vi "Place-cursor.vi"(0 "star X":i16, 1 "GuidePixScale":dbl=0.32, 2 "star Y":i16, 3 "Angle":dbl=0.707, 5 "GuideGraph":refnum<vi>) -> (6 "RA cursor":dbl, 10 "DEC cursor":dbl)   [LabVIEW 2011]
panel:
  in  "camYsize":dbl=480.0
  in  "camXsize":dbl=640.0
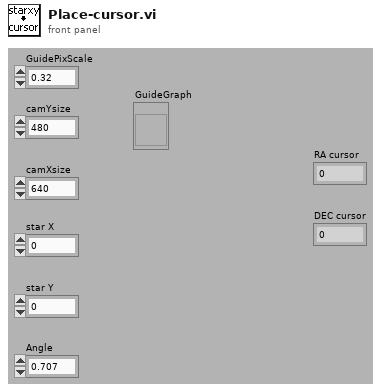
[diagram p1: front panel]
types:
  T1 = typedef "LVRangeTypeDef.ctl" = cluster{"Minimum":dbl, "Maximum":dbl, "Increment":dbl, "Minor Increment":dbl, "Start":dbl}
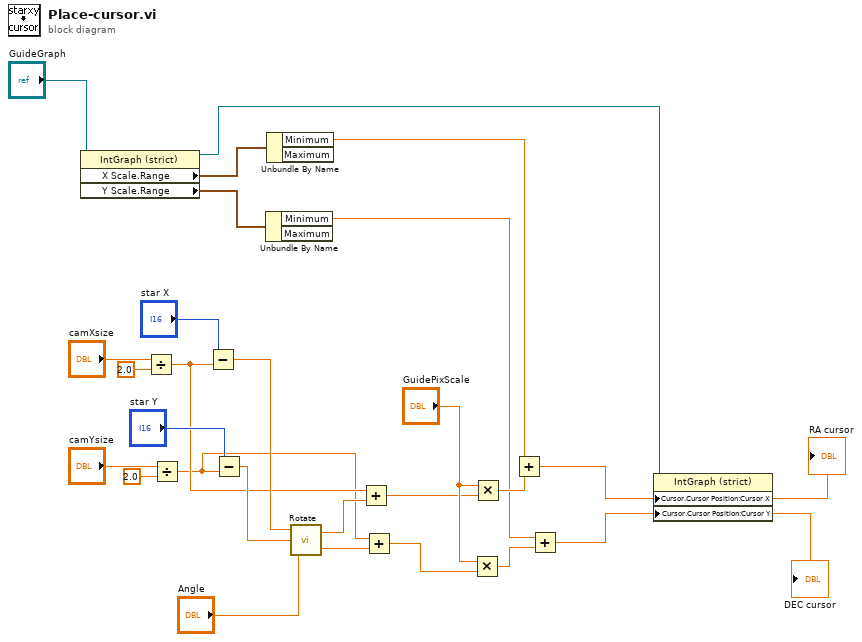
[diagram p0: block diagram]
diagram:
  n1 = property on="Property Node" class="IntGraph (strict)"(reference="GuideGraph") -> (reference out=w10:refnum<vi>, "X Scale.Range"=w18:T1, "Y Scale.Range"=w17:T1)  [unwired: 1 in, 1 out]
  n2 = Divide(x="camXsize", y=2.0) -> (x/y=w7:dbl)
  n3 = Divide(x="camYsize", y=2.0) -> (x/y=w5:dbl)
  n4 = Subtract(x="star X", y=w7) -> (x-y=w19:dbl)
  n5 = Subtract(x="star Y", y=w5) -> (x-y=w20:dbl)
  n6 = Unbundle By Name(w17) -> ("Minimum"=w12:dbl)  [unwired: 1 out]
  n7 = Unbundle By Name(w18) -> ("Minimum"=w13:dbl)  [unwired: 1 out]
  n8 = call "Rotate.vi"("Angle(rad)"="Angle", "Y"=w20, "X"=w19) -> ("rotY"=w4:dbl, "rotX"=w6:dbl)
  n9 = Add(x=w7, y=w6) -> (x+y=w3:dbl)
  n10 = Add(x=w5, y=w4) -> (x+y=w2:dbl)
  n11 = Multiply(x="GuidePixScale", y=w2) -> (x*y=w15:dbl)
  n12 = Multiply(x="GuidePixScale", y=w3) -> (x*y=w16:dbl)
  n13 = Add(x=w13, y=w16) -> (x+y=w9:dbl)
  "RA cursor" <- w9
  n14 = Add(x=w12, y=w15) -> (x+y=w8:dbl)
  "DEC cursor" <- w8
  n15 = property on="Property Node" class="IntGraph (strict)"(reference=w10, "Cursor.Cursor Position:Cursor X"=w9, "Cursor.Cursor Position:Cursor Y"=w8) -> ()  [unwired: 1 in, 2 out]
